vi "Get Sender.vi"(11 "Teardown Msg in":refnum<class "Teardown Msg.lvclass">) -> (2 "Sender":refnum<class "Sender.lvclass">)   [LabVIEW 2020, in "jettl.lvlib" / "Teardown Msg.lvlib" / "Teardown Msg.lvclass"]
uses:
  Teardown Msg.lvclass
  Sender/Sender/Sender.lvclass
  Teardown Msg.lvclass/Teardown Msg.ctl
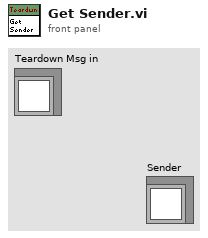
[diagram p1: front panel]
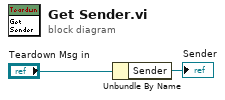
[diagram p0: block diagram]
diagram:
  n1 = Unbundle By Name("Teardown Msg in") -> ("Sender"=→"Sender":refnum<class "Sender.lvclass">)
